vi "Start.vi"(8 "error in (no error)":errorcluster, 11 "Electrophysiology in":refnum<class "AcquireTraces.lvclass">) -> (0 "error out":errorcluster, 3 "Electrophysiology out":refnum<class "AcquireTraces.lvclass">)   [LabVIEW 2014, in "AcquireTraces.lvclass"]
uses:
  AcquireTraces.lvclass
  AcquireTraces.lvclass/AcquireTraces.ctl
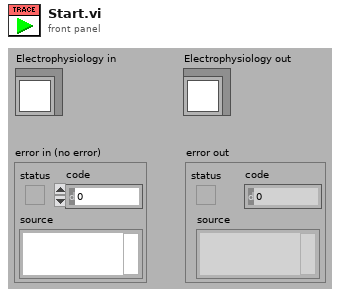
[diagram p1: front panel]
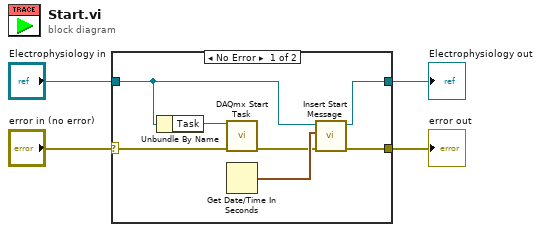
[diagram p0: block diagram]
diagram:
  n1 = case shown="No Error" "error in (no error)" {
    selector: "error in (no error)" -> [w11 w13]
    tunnel: [w6 w13] -> w3
    tunnel: [w5 w12] -> w1
    tunnel: "Electrophysiology in" -> [w9 w12]
    frame No Error {
      n2 = Unbundle By Name(w9) -> ("Task"=w10:refnum<k21>)
      n3 = call <vilib>:"DAQmx Start Task.vi"("task/channels in"=w10, "error in"=w11) -> ("error out"=w7:errorcluster)  [unwired: 12 in, 1 out]
      n4 = Get Date/Time In Seconds() -> (seconds since 1Jan1904=w8:timestamp)
      n5 = call-dynamic "Insert Start Message.vi"("error in (no error)"=w7, "Start Time"=w8, "AcquireTraces in"=w9) -> ("error out"=w6:errorcluster, "AcquireTraces out"=w5:refnum<class "AcquireTraces.lvclass">)  [unwired: 7 in]
    }
    frame Error {
    }
  }
  "error out" <- w3
  "Electrophysiology out" <- w1
